vi "Bob.vi"() -> ()   [LabVIEW 2013]
panel:
  out "Comparação das Bases":string
  out "Bases Alice":string
  out "error out 2":errorcluster
  in  "port":u16
  out "error out":errorcluster
  out "data out":string
  out "Ângulo Servo:":i32
  out "Bases Bob":string
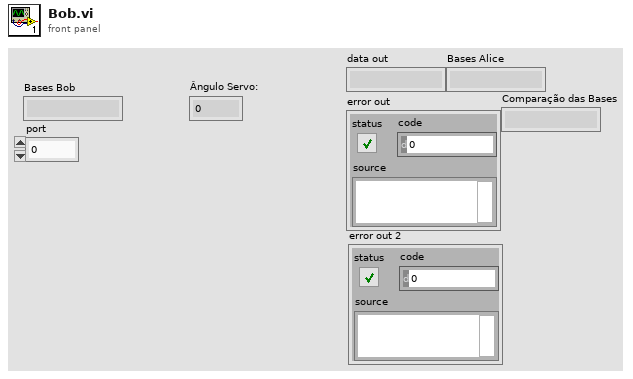
[diagram p1: front panel]
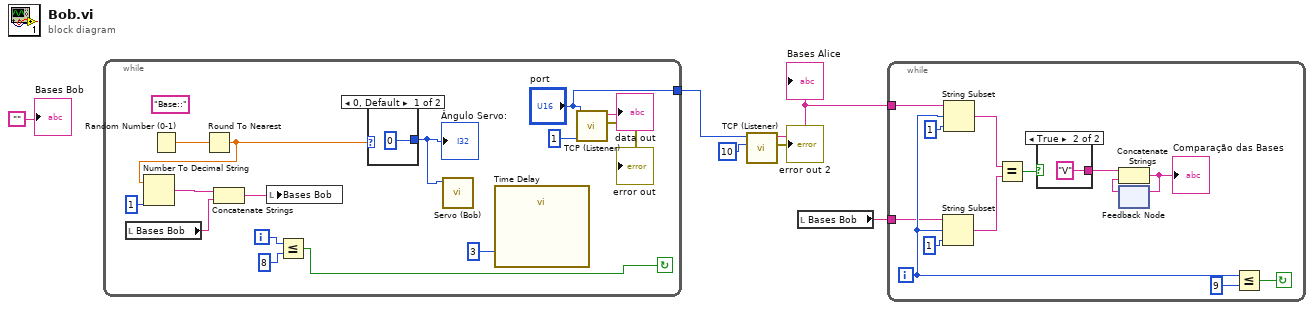
[diagram p0: block diagram]
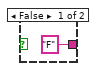
[diagram p2: hidden frame]
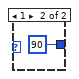
[diagram p3: hidden frame]
diagram:
  n1 = while {
    tunnel: ["port"] -> w6
    i -> [w14]
    stop <- w13 continue-if-true
    (unwired) "Base::"
    n2 = local read "Bases Bob"() -> (w7:string)
    n3 = Random Number (0-1)() -> (number: 0 to 1=w21:dbl)
    n4 = Round To Nearest(number=w21) -> (nearest integer value=w18:dbl)
    n5 = Number To Decimal String(number=w18, width (-)=1) -> (decimal integer string=w19:string)
    n6 = Concatenate Strings(w19, w7) -> (w8:string)
    n7 = local write "Bases Bob"(w8) -> ()
    n8 = Less Or Equal?(x=w14, y=8) -> (x <= y?=w13:bool)
    n9 = case shown="0, Default" w18 {
      tunnel: [0 90] -> w17
      frame 0, Default {
      }
      frame 1 {
      }
    }
    "Ângulo Servo:" <- w17
    n10 = call "Servo (Bob).vi"("Ângulo Servo:"=w17) -> ()  [unwired: 11 in]
    n11 = call "Time Delay"("Delay Time (s)"=3) -> ()  [unwired: 10 in, 1 out]
    n12 = call "TCP (Listener).vi"("bytes to read"=1, "port"="port") -> ("error out"=→"error out":errorcluster, "data out"=→"data out":string)  [unwired: 8 in]
  }
  n13 = call "TCP (Listener).vi"("bytes to read"=10, "port"=w6) -> ("error out"=→"error out 2":errorcluster, "data out"=w3:string)  [unwired: 8 in]
  "Bases Alice" <- w3
  n14 = local read "Bases Bob"() -> (w2:string)
  n15 = while {
    tunnel: w3 -> [w36]
    tunnel: w2 -> [w24]
    i -> [w25]
    stop <- w32 continue-if-true
    n16 = String Subset(string=w24, offset (0)=w25, length (rest)=1 ("length (rest)")) -> (substring=w30:string)
    n17 = String Subset(string=w36, offset (0)=w25, length (rest)=1 ("length (rest)")) -> (substring=w31:string)
    n18 = Equal?(x=w31, y=w30) -> (x = y?=w29:bool)
    n19 = case shown="True" w29 {
      tunnel: ["F" "V"] -> w28
      frame False {
      }
      frame True {
      }
    }
    n20 = feedback #1() -> (w26:string)  [unwired: 1 in]
    n21 = Concatenate Strings(w28, w26) -> (w27:string)
    "Comparação das Bases" <- w27
    n22 = feedback-in #1(w27) -> ()
    n23 = Less Or Equal?(x=w25, y=9) -> (x <= y?=w32:bool)
  }
  "Bases Bob" <- ""
